vi "util-timestring-to-timestamp.vi"(8 "error in":errorcluster, 11 "String Value":string) -> (0 "error out":errorcluster, 3 "Time Stamp":timestamp)   [LabVIEW 2024]
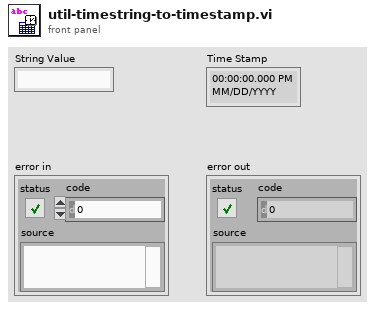
[diagram p1: front panel]
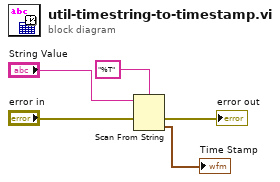
[diagram p0: block diagram]
diagram:
  n1 = Scan From String(format string="%T", input string="String Value", error in="error in") -> (error out=→"error out":errorcluster, output 1=→"Time Stamp":timestamp)  [unwired: 2 in, 2 out]
